vi "VPA QC Leak Test.vi"(7 "DAQ Q":T1, 9 "DAQ Ref Cluster":T2, 10 "State Cluster":T3) -> (2 "State Cluster Out":T3)   [LabVIEW 2013]
uses:
  Controls/VPA QC State Data Cluster.ctl
  Controls/VPA QC General Cluster.ctl
  Controls/VPA QC State Enum.ctl
  Controls/VPA QC Bool Cluster.ctl
  Controls/VPA QC DAQ Ref Cluster.ctl
  Controls/VPA QC DAQ Q.ctl
  Controls/VPA QC DAQ Cmd Enum.ctl
panel:
  out "DAQ Error Msg":string
  in  "Cancel":bool
  in  "Save":bool
  in  "Cancel Logging":bool
  out "Time Remaining":dbl
  in  "Log":bool
  in  "Close Valves":bool
  out "Manifold Leak Test":dbl[][](graph)
  # "Manifold/Cylinder Leak Test"
  # "1. In pressure control mode, ramp to 95% max pressure."
  # "2. Close all manifold valves"
  # "3. Stop pressure control"
  # "4. Open External Valve. Record the pressure in the table below for 10 minutes."
  # "5. Start logging the pressure."
  # "Assembly Checklist"
  # "Assembly Checklist"
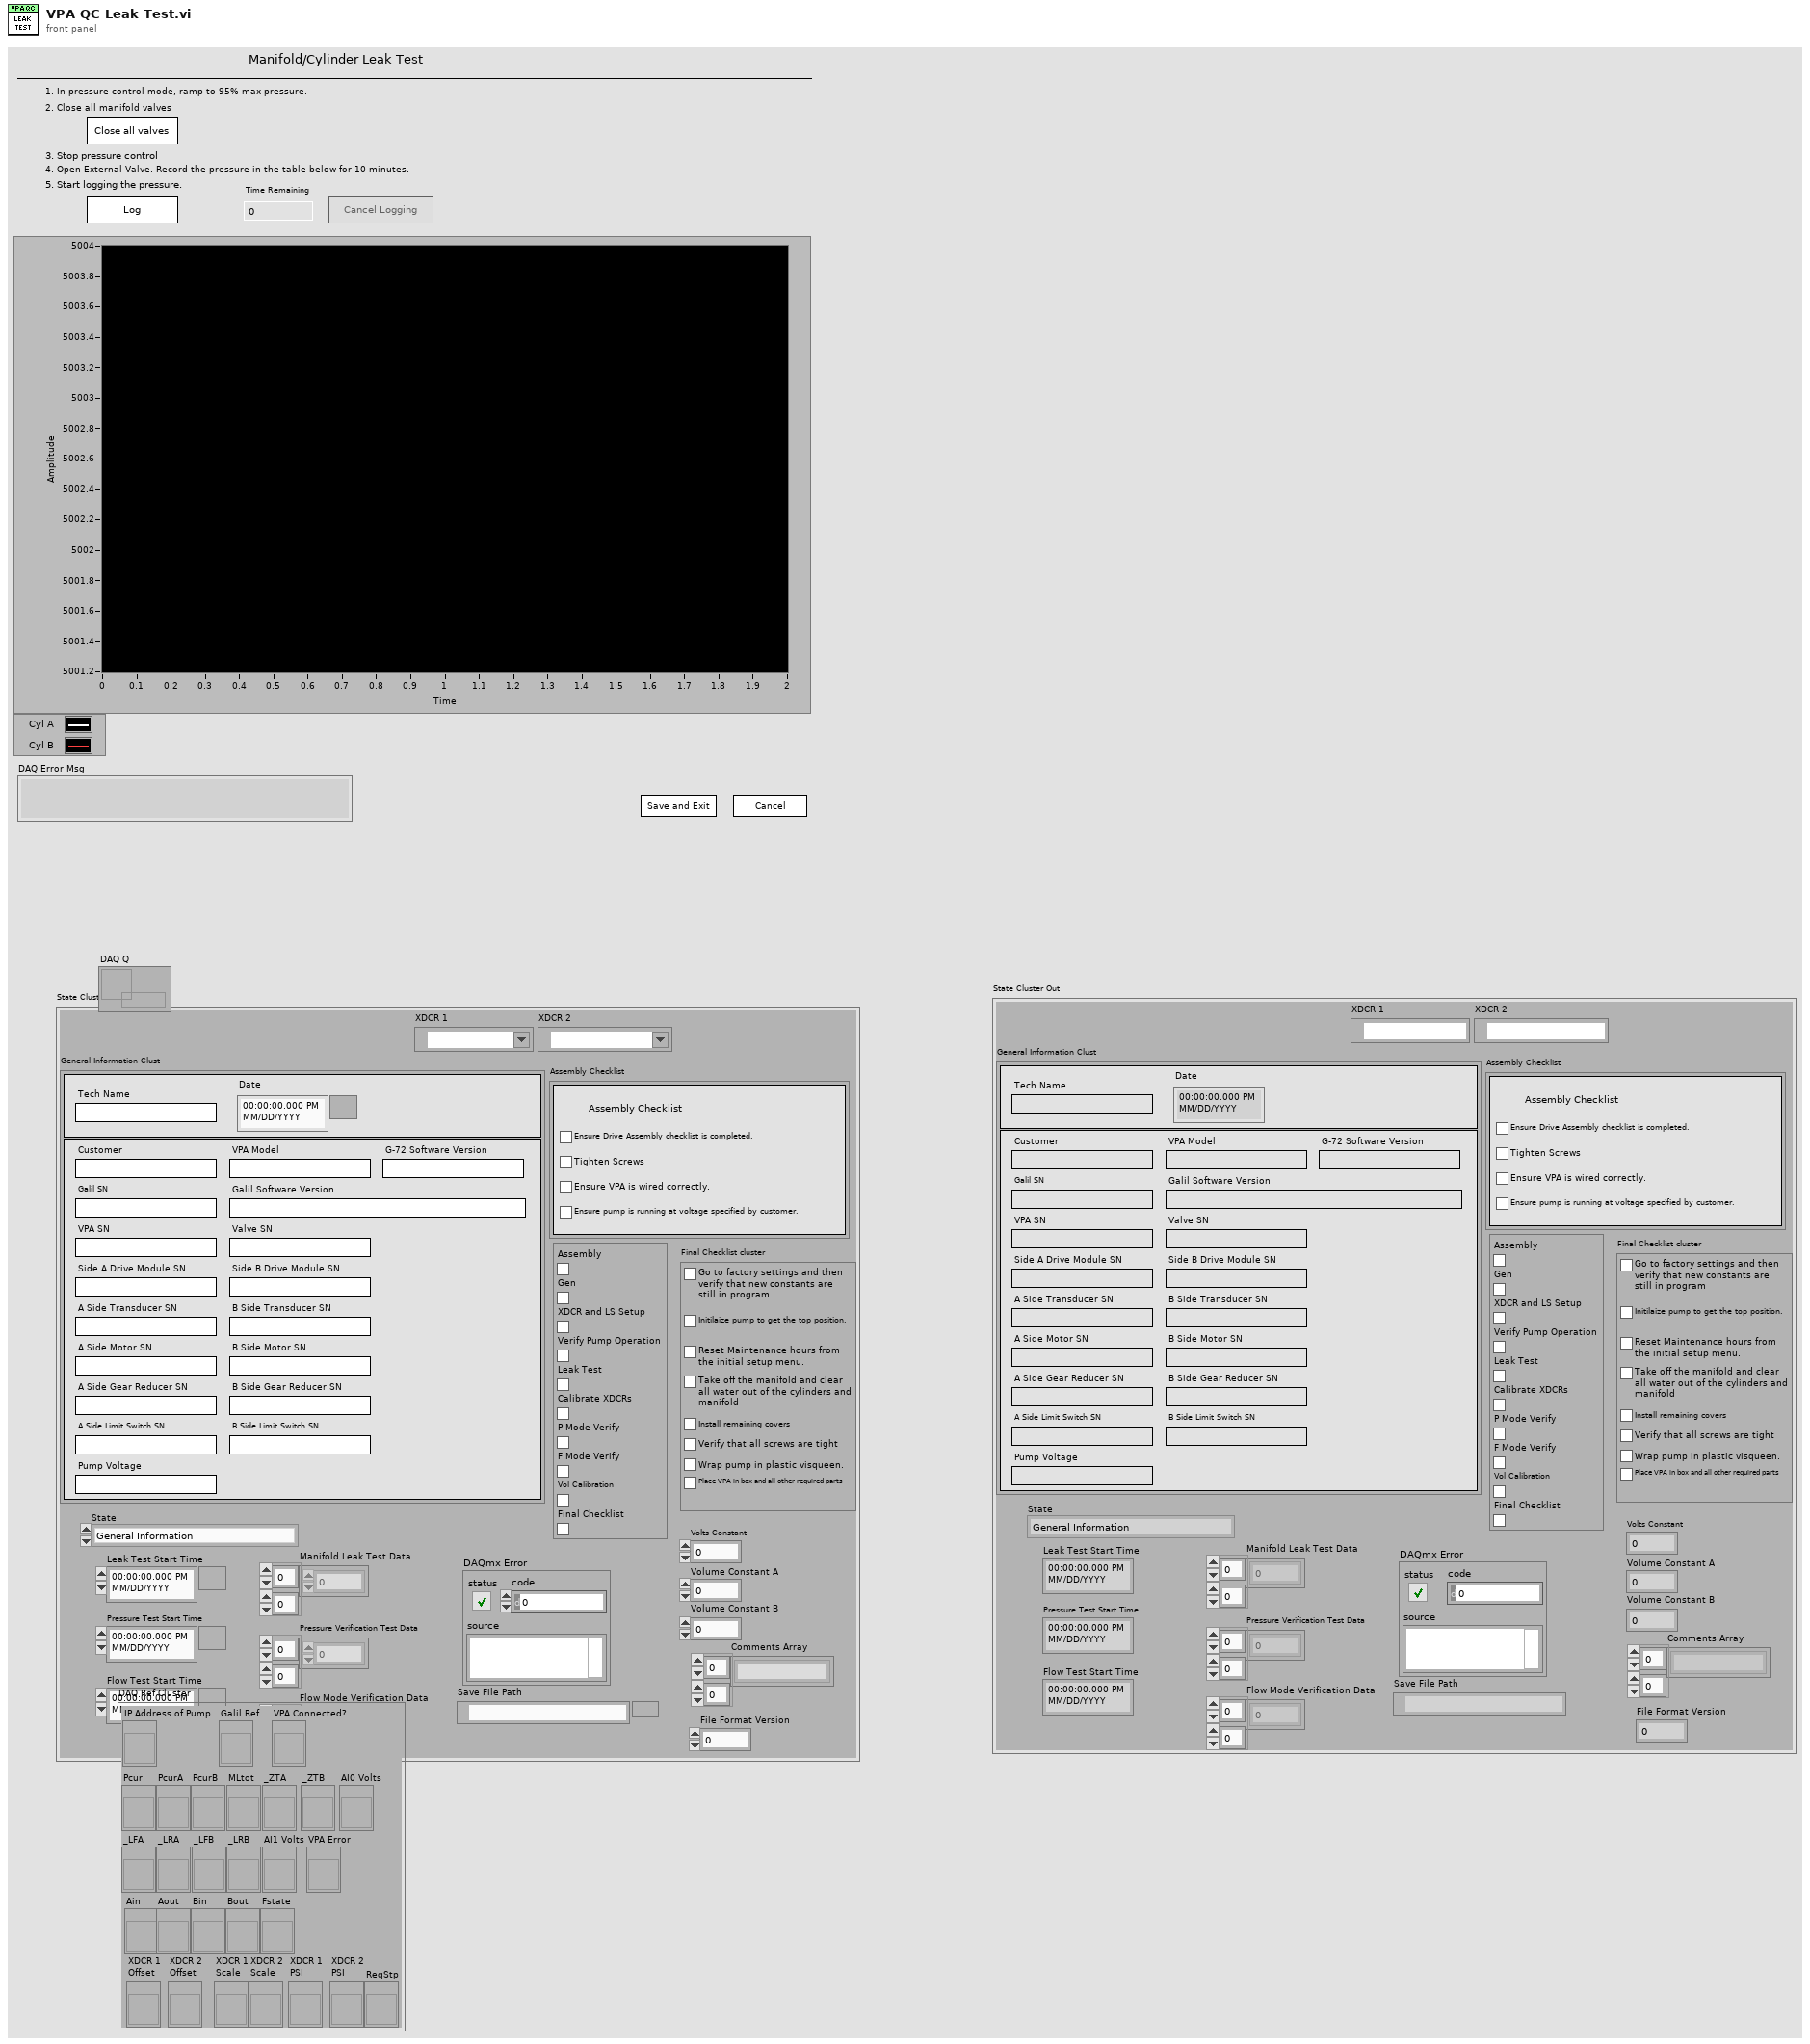
[diagram p1: front panel]
types:
  T1 = typedef "VPA QC DAQ Q.ctl" = refnum<queue>
  T2 = typedef "VPA QC DAQ Ref Cluster.ctl" = cluster{"IP Address of Pump":refnum<vi>, "Galil Ref":refnum<vi>, "VPA Connected?":refnum<vi>, "Pcur":refnum<vi>, "PcurA":refnum<vi>, "PcurB":refnum<vi>, "MLtot":refnum<vi>, "_LFA":refnum<vi>, "_LRA":refnum<vi>, "_LFB":refnum<vi>, "_LRB":refnum<vi>, "_ZTA":refnum<vi>, "_ZTB":refnum<vi>, "AI0 Volts":refnum<vi>, "AI1 Volts":refnum<vi>, "VPA Error":refnum<vi>, "Ain":refnum<vi>, "Aout":refnum<vi>, "Bin":refnum<vi>, "Bout":refnum<vi>, "Fstate":refnum<vi>, "XDCR 1\nOffset":refnum<vi>, "XDCR 2 \nOffset":refnum<vi>, "XDCR 1\nScale":refnum<vi>, "XDCR 2\nScale":refnum<vi>, "XDCR 1\nPSI":refnum<vi>, "XDCR 2\nPSI":refnum<vi>, "ReqStp":refnum<vi>}
  T3 = typedef "VPA QC State Data Cluster.ctl" = cluster{"XDCR 1":tag, "XDCR 2":tag, "General Information Clust":T4, "Assembly Checklist":cluster{"Ensure Drive Assembly checklist is completed.":bool, "Tighten Screws":bool, "Ensure VPA is wired correctly.":bool, "Ensure pump is running at voltage specified by customer.":bool}, "State":T5, "Manifold Leak Test Data":dbl[][], "Pressure Verification Test Data":dbl[][], "Flow Mode Verification Data":dbl[][], "DAQmx Error":errorcluster, "Bool Cluster":T6, "Leak Test Start Time":timestamp, "Pressure Test Start Time":timestamp, "Flow Test Start Time":timestamp, "Final Checklist cluster":cluster{"Check Fact Rest":bool, "Initialize Pump":bool, "Maintenance Hours":bool, "Clean Water Out":bool, "Covers":bool, "Screws":bool, "Wrap":bool, "Box":bool}, "Volts Constant":dbl, "Volume Constant A":dbl, "Volume Constant B":dbl, "Save File Path":path, "Comments Array":string[][], "File Format Version":u16}
  T4 = typedef "VPA QC General Cluster.ctl" = cluster{"Tech Name":string, "Date":timestamp, "Customer":string, "VPA Model":string, "G-72 Software Version":string, "Galil SN":string, "Galil Software Version":string, "VPA SN":string, "Valve SN":string, "Side A Drive Module SN":string, "Side B Drive Module SN":string, "A Side Transducer SN":string, "B Side Transducer SN":string, "A Side Motor SN":string, "B Side Motor SN":string, "A Side Gear Reducer SN":string, "B Side Gear Reducer SN":string, "A Side Limit Switch SN":string, "B Side Limit Switch SN":string, "Pump Voltage":string}
  T5 = typedef "VPA QC State Enum.ctl" = enum16{"General Information", "XDCR and LS Check", "Check Pump Function", "Manifold/Cylinder Leak Test", "Exit"}
  T6 = typedef "VPA QC Bool Cluster.ctl" = cluster{"Assembly":bool, "Gen":bool, "XDCR and LS Setup":bool, "Verify Pump Operation":bool, "Leak Test":bool, "Calibrate XDCRs":bool, "P Mode Verify":bool, "F Mode Verify":bool, "Vol Calibration":bool, "Final Checklist":bool}
  T7 = enum8{"Enabled", "Disabled", "Disabled and Grayed Out"}
  T8 = typedef "VPA QC DAQ Cmd Enum.ctl" = enum16{"Connect", "Disconnect", "Quit", "Close All Valves", "Burn Calibration"}
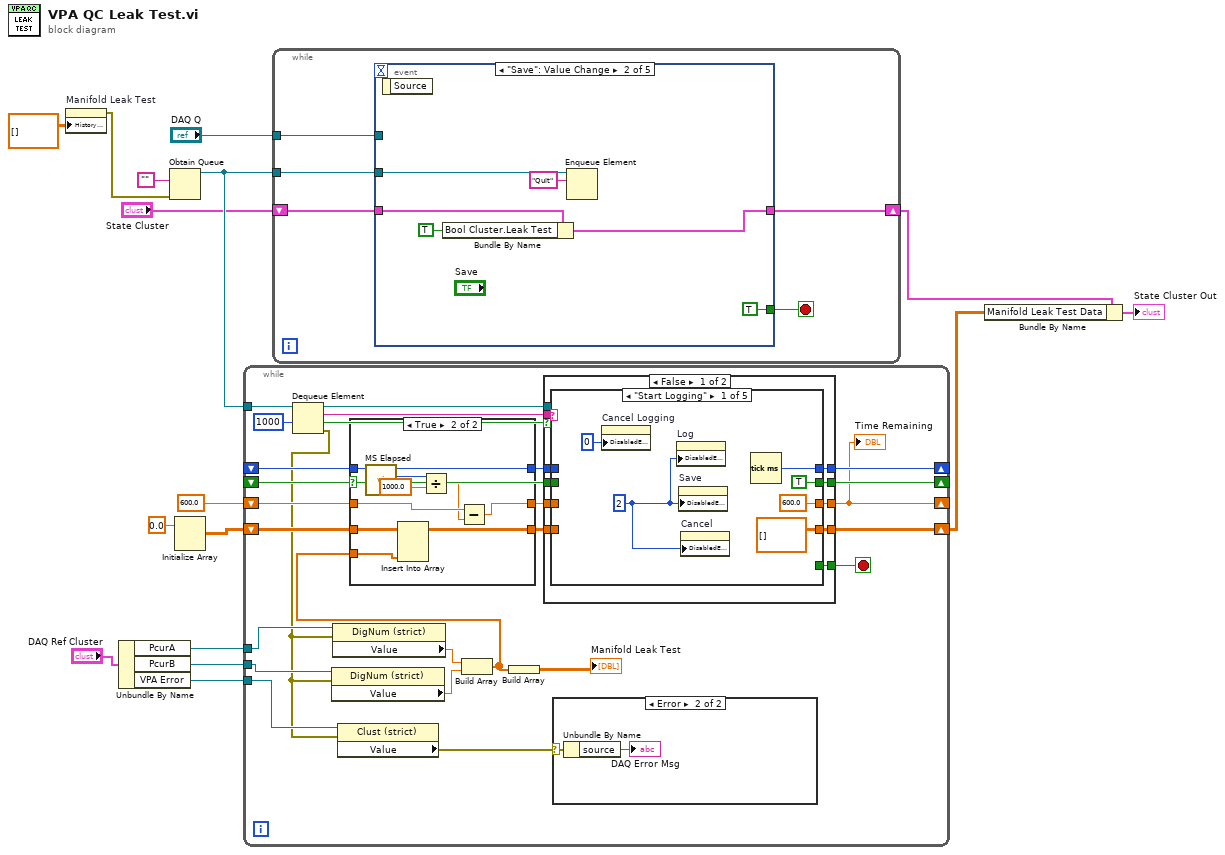
[diagram p0: block diagram]
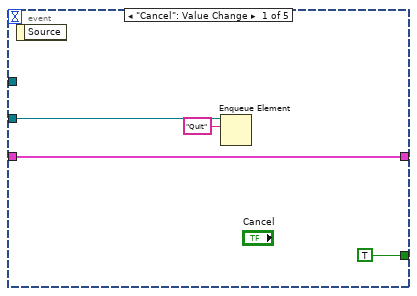
[diagram p2: hidden frame]
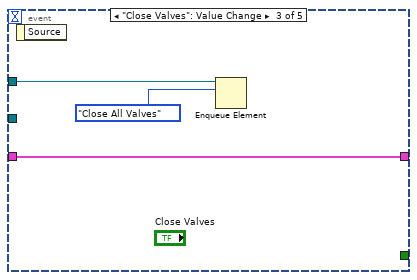
[diagram p3: hidden frame]
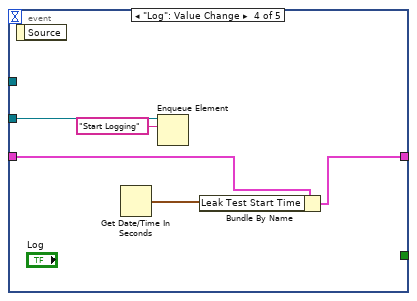
[diagram p4: hidden frame]
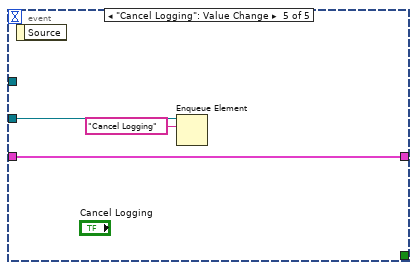
[diagram p5: hidden frame]
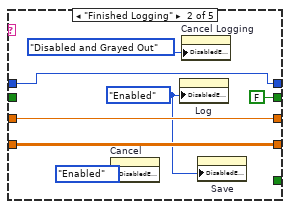
[diagram p8: hidden frame]
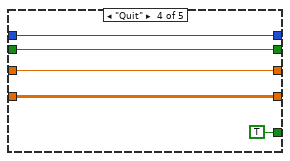
[diagram p10: hidden frame]
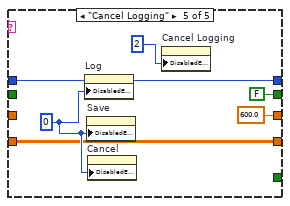
[diagram p11: hidden frame]
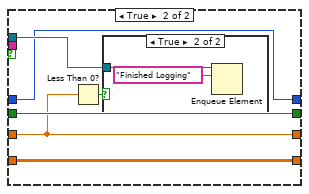
[diagram p12: hidden frame]
diagram:
  n1 = property on="Manifold Leak Test" class="WFChart (strict)"("History Data"=dbl[][] [] ("Manifold Leak Test")) -> (error out=w1:errorcluster)  [unwired: 2 in, 1 out]
  n2 = Unbundle By Name("DAQ Ref Cluster") -> ("PcurA"=w15:refnum<vi>, "PcurB"=w14:refnum<vi>, "VPA Error"=w4:refnum<vi>)
  n3 = Obtain Queue(element data type="", error in (no error)=w1) -> (queue out=w12:refnum<queue>)  [unwired: 3 in, 2 out]
  n4 = Initialize Array(0.0 ("element")) -> (w11:dbl[][])  [unwired: 2 in]
  n5 = while {
    tunnel: w15 -> [w41]
    tunnel: w14 -> [w42]
    tunnel: w12 -> [w38]
    shift-right: [w33] -> _
    shift-left: _ -> [w31]
    shift-right: [w29] -> w3
    shift-left: w11 -> [w32]
    shift-right: [w22] -> _
    shift-left: 600.0 -> [w28]
    shift-right: [w23] -> _
    shift-left: _ -> [w25]
    tunnel: w4 -> [w21]
    stop <- w34 stop-if-true
    n6 = Dequeue Element(queue=w38, timeout in ms (-1)=1000) -> (queue out=w26:refnum<queue>, element=w36:string, timed out?=w35:bool, error out=w19:errorcluster)  [unwired: 1 in]
    n7 = property class="DigNum (strict)"(reference=w42, error in=w19) -> ("Value"=w39:dbl)  [unwired: 2 out]
    n8 = property class="DigNum (strict)"(reference=w41, error in=w19) -> ("Value"=w40:dbl)  [unwired: 2 out]
    n9 = property class="Clust (strict)"(reference=w21, error in=w19) -> ("Value"=w20:errorcluster)  [unwired: 2 out]
    n10 = Build Array(w40, w39) -> (w17:dbl[])
    n11 = case shown="True" w31 {
      tunnel: w17 -> [_ w56]
      tunnel: w32 -> [w47 w57]
      tunnel: [w47 w55] -> w30
      tunnel: w28 -> [w46 w54]
      tunnel: [w46 w53] -> w27
      tunnel: w25 -> [w45 w49]
      tunnel: [w45 w48] -> w24
      frame False {
      }
      frame True {
        n12 = call "MS Elapsed.vi"("ms in"=w49) -> ("elapsed ms"=w52:u32, "new ms time"=w48:u32)  [unwired: 9 in]
        n13 = Insert Into Array(array=w57, new element=w56) -> (w55:dbl[][])  [unwired: 2 in]
        n14 = Divide(x=w52, y=1000.0) -> (x/y=w50:dbl)
        n15 = Subtract(x=w54, y=w50) -> (x-y=w53:dbl)
      }
    }
    n16 = Build Array(w17) -> (→"Manifold Leak Test":dbl[][])
    n17 = case shown="False" w35 {
      tunnel: w36 -> [w67 _]
      tunnel: [w66 _] -> w34
      tunnel: [w65 w101] -> w33
      tunnel: w31 -> [w64 w101]
      tunnel: w30 -> [w63 w100]
      tunnel: [w62 w100] -> w29
      tunnel: w27 -> [w61 w99]
      tunnel: [w60 w99] -> w22
      tunnel: w26 -> [_ w97]
      tunnel: w24 -> [w59 w96]
      tunnel: [w58 w96] -> w23
      frame False {
        n18 = case shown="\"Start Logging\"" w67 {
          tunnel: [_ _ _ TRUE _] -> w66
          tunnel: [TRUE FALSE w84 w88 FALSE] -> w65
          tunnel: w64 -> [_ _ w84 w88 _]
          tunnel: w63 -> [_ w80 w83 w87 w90]
          tunnel: [dbl[][] [] w80 w83 w87 w90] -> w62
          tunnel: w61 -> [_ w79 w82 w86 _]
          tunnel: [600.0 w79 w82 w86 600.0] -> w60
          tunnel: w59 -> [_ w74 w81 w85 w93]
          tunnel: [w71 w74 w81 w85 w93] -> w58
          frame "Start Logging" {
            w69 = u8 2
            n19 = property on="Cancel Logging" class="Bool"("DisabledEnum"=u8 0) -> ()  [unwired: 2 in, 2 out]
            n20 = property on="Log" class="Bool"("DisabledEnum"=w69) -> ()  [unwired: 2 in, 2 out]
            n21 = property on="Save" class="Bool"("DisabledEnum"=w69) -> ()  [unwired: 2 in, 2 out]
            n22 = property on="Cancel" class="Bool"("DisabledEnum"=w69) -> ()  [unwired: 2 in, 2 out]
            n23 = Tick Count (ms)() -> (millisecond timer value=w71:u32)
          }
          frame "Finished Logging" {
            w75 = T7."Enabled" ("Disabled")
            n24 = property on="Cancel" class="Bool"("DisabledEnum"=T7."Enabled" ("Disabled")) -> ()  [unwired: 2 in, 2 out]
            n25 = property on="Log" class="Bool"("DisabledEnum"=w75) -> ()  [unwired: 2 in, 2 out]
            n26 = property on="Cancel Logging" class="Bool"("DisabledEnum"=T7."Disabled and Grayed Out" ("Disabled")) -> ()  [unwired: 2 in, 2 out]
            n27 = property on="Save" class="Bool"("DisabledEnum"=w75) -> ()  [unwired: 2 in, 2 out]
          }
          frame Default {
          }
          frame "Quit" {
          }
          frame "Cancel Logging" {
            w92 = u8 0
            n28 = property on="Log" class="Bool"("DisabledEnum"=w92) -> ()  [unwired: 2 in, 2 out]
            n29 = property on="Save" class="Bool"("DisabledEnum"=w92) -> ()  [unwired: 2 in, 2 out]
            n30 = property on="Cancel" class="Bool"("DisabledEnum"=w92) -> ()  [unwired: 2 in, 2 out]
            n31 = property on="Cancel Logging" class="Bool"("DisabledEnum"=u8 2) -> ()  [unwired: 2 in, 2 out]
          }
        }
      }
      frame True {
        n32 = Less Than 0?(x=w99) -> (x < 0?=w98:bool)
        n33 = case shown="True" w98 {
          tunnel: w97 -> [_ w103]
          frame False {
          }
          frame True {
            n34 = Enqueue Element(queue=w103, element="Finished Logging") -> ()  [unwired: 2 in, 3 out]
          }
        }
      }
    }
    "Time Remaining" <- w22
    n35 = case shown="Error" w20 {
      selector: w20 -> [_ w44]
      frame No Error {
      }
      frame Error {
        n36 = Unbundle By Name(w44) -> ("source"=→"DAQ Error Msg":string)
      }
    }
  }
  n37 = while {
    tunnel: w12 -> [w107]
    shift-right: [w105] -> w6
    shift-left: "State Cluster" -> [w106]
    tunnel: "DAQ Q" -> [w104]
    stop <- w108 stop-if-true
    n38 = event shown="[1] \"Save\": Value Change" {
      selector: _ -> [_ _ _ _ _]
      dyn-events: _ -> [_ _ _ _ _]
      timeout: _ -> [_ _ _ _ _]
      tunnel: [TRUE TRUE _ _ _] -> w108
      tunnel: w107 -> [w111 w114 _ w126 w129]
      tunnel: w106 -> [w109 w117 w121 w123 w127]
      tunnel: [w109 w115 w121 w122 w127] -> w105
      tunnel: w104 -> [_ _ w120 _ _]
      event "Cancel": Value Change {
        n39 = event-data() -> ()  [unwired: 1 in, 1 out]
        n40 = Enqueue Element(queue=w111, element="Quit") -> ()  [unwired: 2 in, 3 out]
      }
      event "Save": Value Change {
        n41 = event-data() -> ()  [unwired: 1 in, 1 out]
        n42 = Bundle By Name(cluster=w117, "Bool Cluster.Leak Test"=TRUE) -> (w115:T3)
        n43 = Enqueue Element(queue=w114, element="Quit") -> ()  [unwired: 2 in, 3 out]
      }
      event "Close Valves": Value Change {
        n44 = event-data() -> ()  [unwired: 1 in, 1 out]
        n45 = Enqueue Element(queue=w120, element=VPA_QC_DAQ_Cmd_Enum."Close All Valves" ("DAQ loop cmd")) -> ()  [unwired: 2 in, 3 out]
      }
      event "Log": Value Change {
        n46 = event-data() -> ()  [unwired: 1 in, 1 out]
        n47 = Get Date/Time In Seconds() -> (seconds since 1Jan1904=w124:timestamp)
        n48 = Enqueue Element(queue=w126, element="Start Logging") -> ()  [unwired: 2 in, 3 out]
        n49 = Bundle By Name(cluster=w123, "Leak Test Start Time"=w124) -> (w122:T3)
      }
      event "Cancel Logging": Value Change {
        n50 = event-data() -> ()  [unwired: 1 in, 1 out]
        n51 = Enqueue Element(queue=w129, element="Cancel Logging") -> ()  [unwired: 2 in, 3 out]
      }
    }
  }
  n52 = Bundle By Name(cluster=w6, "Manifold Leak Test Data"=w3) -> (→"State Cluster Out":T3)
